vi "CONFOCAL MICROSCOPE - ( POSITION CURSOR).vi"() -> ()   [LabVIEW 2025]
uses:
  <vilib>/Analysis/1siggen.llb/Ramp Pattern by Samples.vi
  <vilib>/DAQmx/write.llb/DAQmx Write (Analog 1D Wfm NChan NSamp).vi
  <vilib>/DAQmx/read.llb/DAQmx Read (Counter 1D U32 1Chan NSamp).vi
  <vilib>/DAQmx/create/channels.llb/DAQmx Create Channel (AO-Voltage-Basic).vi
  <vilib>/DAQmx/configure/timing.llb/DAQmx Timing (Sample Clock).vi
  <vilib>/DAQmx/configure/events/hardwareSignals.llb/DAQmx Export Signal (Most Signals).vi
  <vilib>/DAQmx/miscellaneous.llb/DAQmx Fill In Error Info.vi
  <vilib>/DAQmx/create/channels.llb/DAQmx Create Channel (CI-Count Edges).vi
  <vilib>/Analysis/NI_AALBase.lvlib
panel:
  out "64bit integer":i64[](array[numeric])
  in  "volts":dbl=1.0 format="%_2f"
  in  "pixels":dbl
  out "transposed array":dbl[][](array[numeric])
  out "Intensity Graph":dbl[][](graph)
  out "Min Voltage (V)":dbl
  out "Max Voltage (V)":dbl
  in  "Dwell time (s)":dbl
  in  "Sample mode":i32(ring)=10178 items=["Finite Samples"=10178, "Continuous Samples"=10123, "Hardware Timed Single Point"=12522]
  out "appended array":dbl[][](array[numeric])
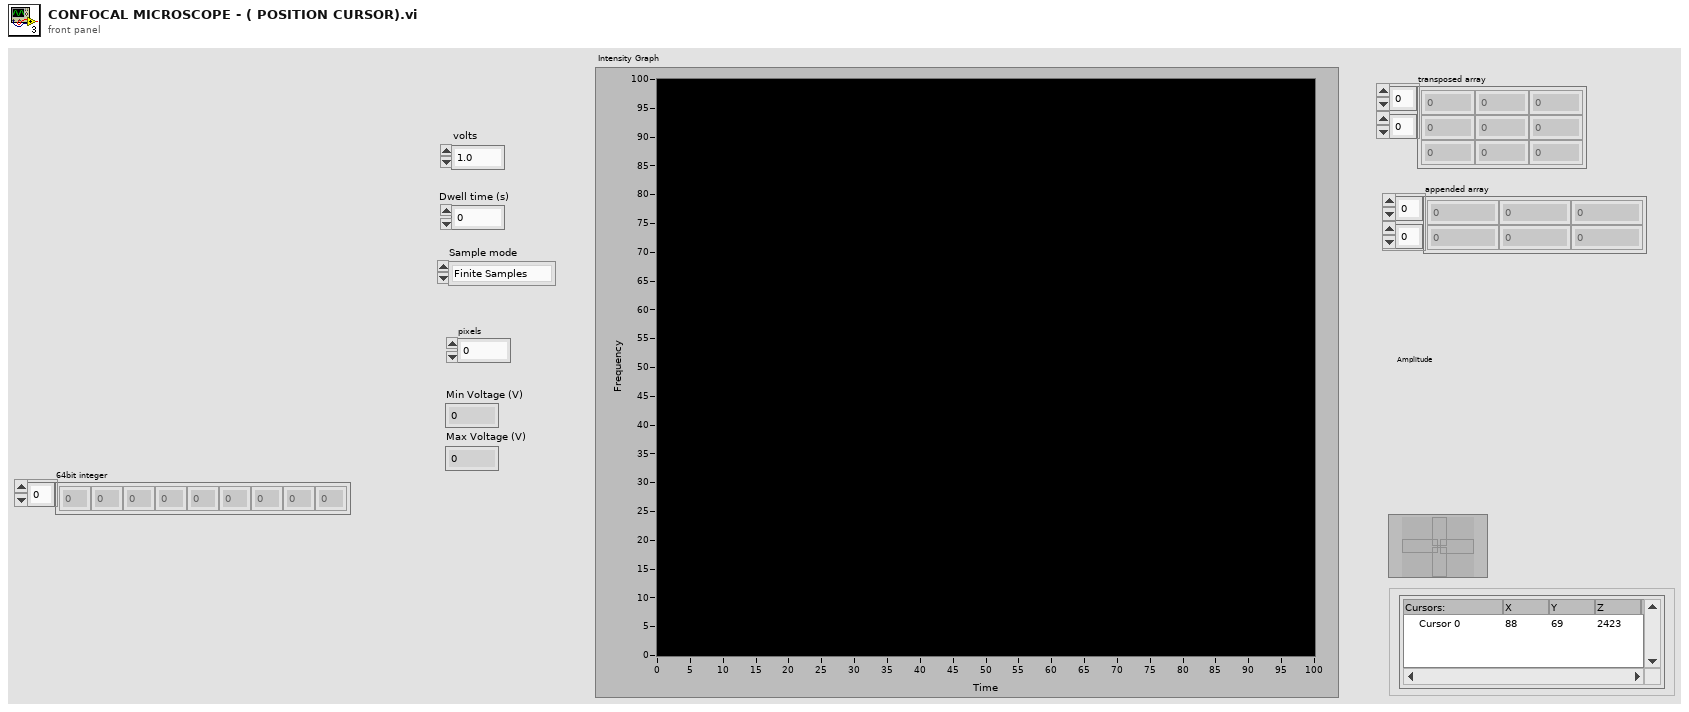
[diagram p1: front panel]
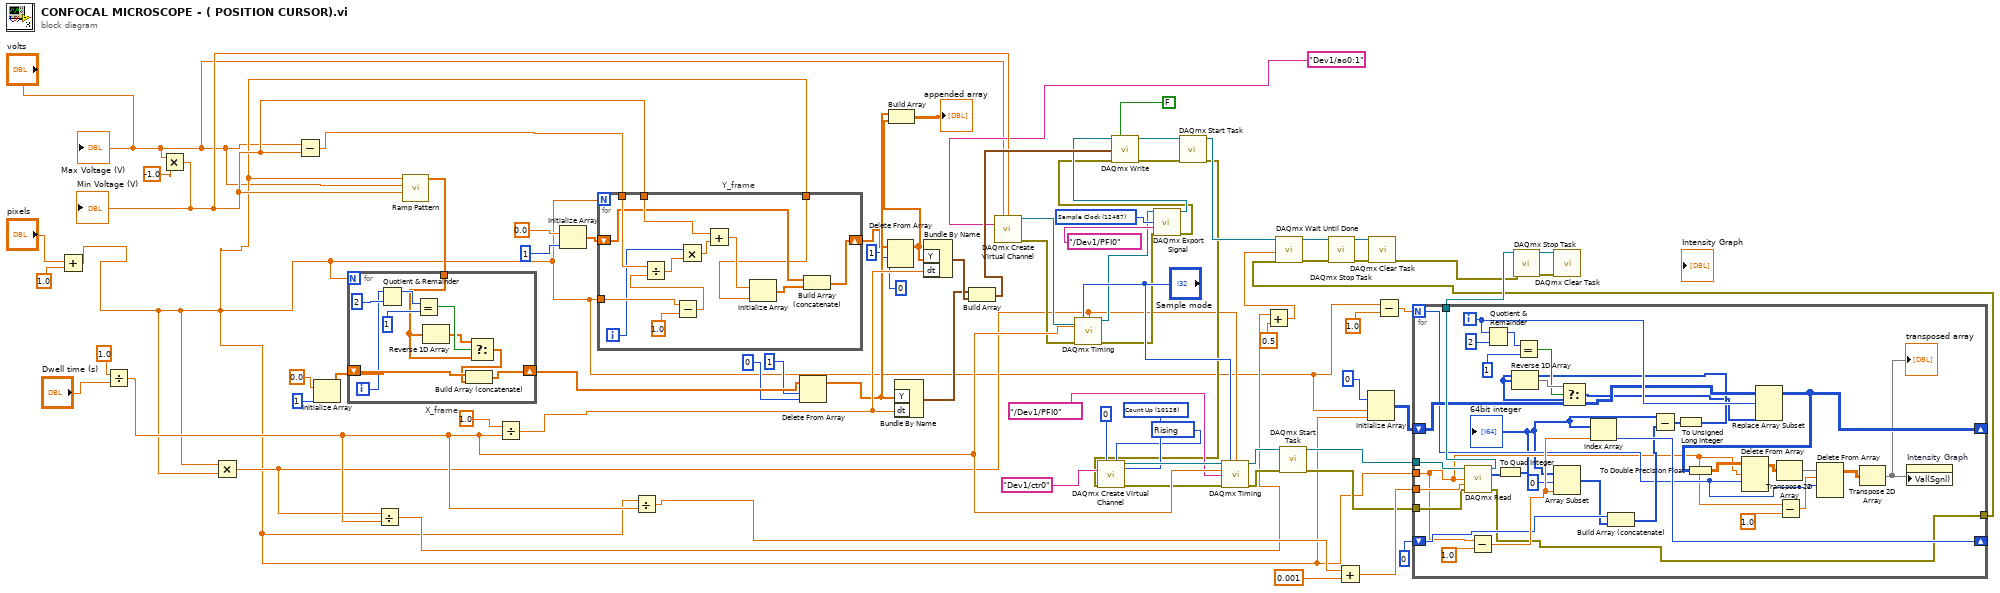
[diagram p0: block diagram]
diagram:
  w45 = 12487 items=["AI Convert Clock"=12484, "10MHz Reference Clock"=12536, "20MHz Timebase Clock"=12486, "Sample Clock"=12487, "Advance Trigger"=12488, "Reference Trigger"=12490, "Start Trigger"=12491, "Advance Complete Event"=12492, "AI Hold Complete Event"=12493, "Counter Output Event"=12494, "Change Detection Event"=12511, "Watchdog Timer Expired Event"=12512] ("signal")
  w50 = 10280 items=["Rising"=10280, "Falling"=10171] ("edge")
  w51 = 10128 items=["Count Up"=10128, "Count Down"=10124, "Externally Controlled"=10326] ("count direction")
  n1 = Add(x="pixels", y=1.0) -> (x+y=w2:dbl)
  n2 = Divide(x=1.0, y="Dwell time (s)") -> (x/y=w30:dbl)
  n3 = Multiply(x="volts", y=-1.0) -> (x*y=w6:dbl)
  "Min Voltage (V)" <- w6
  n4 = Multiply(x=w2, y=w2) -> (x*y=w11:dbl)
  n5 = Subtract(x="volts", y=w6) -> (x-y=w47:dbl)
  n6 = Initialize Array(0.0 ("element"), 1 ("dimension size")) -> (w58:dbl[])
  n7 = Divide(x=w11, y=w30) -> (x/y=w10:dbl)
  n8 = call-poly <vilib>:"Ramp Pattern.vi"("start"=w6, "end"="volts", "samples"=w2) -> ("Ramp Pattern"=w74:dbl[])  [unwired: 7 in, 1 out]
  n9 = for "X_frame" {
    N: w2 -> [_]
    shift-right: [w87] -> w41
    shift-left: w58 -> [w88]
    tunnel: w74 -> [w81]
    i -> [w82]
    n10 = Quotient & Remainder(x=w82, y=2) -> (x-y*floor(x/y)=w85:i32)  [unwired: 1 out]
    n11 = Equal?(x=w85, y=1) -> (x = y?=w83:bool)
    n12 = Reverse 1D Array(array=w81) -> (reversed array=w80:dbl[])
    n13 = Select(t=w80, s=w83, f=w81) -> (s? t:f=w79:dbl[])
    n14 = Build Array (concatenate)(w88, w79) -> (w87:dbl[])
  }
  n15 = Divide(x=1.0, y=w30) -> (x/y=w60:dbl)
  n16 = Initialize Array(0.0 ("element"), 1 ("dimension size")) -> (w59:dbl[])
  n17 = for "Y_frame" {
    N: w2 -> [_]
    tunnel: w2 -> [w101]
    tunnel: w47 -> [w99]
    tunnel: w6 -> [w94]
    tunnel: w2 -> [w89]
    shift-right: [w90] -> w37
    shift-left: w59 -> [w91]
    i -> [w96]
    n18 = Subtract(x=w101, y=1.0) -> (x-y=w98:dbl)
    n19 = Divide(x=w99, y=w98) -> (x/y=w97:dbl)
    n20 = Multiply(x=w96, y=w97) -> (x*y=w95:dbl)
    n21 = Add(x=w94, y=w95) -> (x+y=w93:dbl)
    n22 = Initialize Array(w93, w89) -> (w92:dbl[])
    n23 = Build Array (concatenate)(w91, w92) -> (w90:dbl[])
  }
  n24 = Divide(x=w2, y=w30) -> (x/y=w26:dbl)
  n25 = Delete From Array "Delete From Array"(array=w41, length=1, index=0) -> (array with subset deleted=w38:dbl[])  [unwired: 1 out]
  n26 = Delete From Array "Delete From Array"(array=w37, length=1, index=0) -> (array with subset deleted=w31:dbl[])  [unwired: 1 out]
  n27 = Build Array(w38, w31) -> (→"appended array":dbl[][])
  n28 = Bundle By Name("Y"=w38, "dt"=w60) -> (w61:waveform(dbl))  [unwired: 1 in]
  n29 = Bundle By Name("Y"=w31, "dt"=w60) -> (w62:waveform(dbl))  [unwired: 1 in]
  n30 = Build Array(w61, w62) -> (w64:waveform(dbl)[])
  n31 = call-poly <vilib>:"DAQmx Create Virtual Channel.vi"("maximum value"="volts", "minimum value"=w6, "physical channels"="Dev1/ao0:1" ("Galvo mirror path")) -> ("task out"=w63:refnum<k21>, "error out"=w24:errorcluster)  [unwired: 11 in]
  n32 = call-poly <vilib>:"DAQmx Timing.vi"("task/channels in"=w63, "sample mode"="Sample mode", "samples per channel"=w11, "rate"=w30, "error in"=w24) -> ("task out"=w43:refnum<k21>, "error out"=w23:errorcluster)  [unwired: 9 in]
  n33 = call-poly <vilib>:"DAQmx Export Signal.vi"("task/channels in"=w43, "signal"=w45, "output terminal"=tag "/Dev1/PFI0", "error in"=w23) -> ("task out"=w42:refnum<k21>, "error out"=w22:errorcluster)  [unwired: 10 in]
  n34 = call-poly <vilib>:"DAQmx Write.vi"("task/channels in"=w42, "auto start"=FALSE, "data"=w64, "error in"=w22) -> ("task out"=w65:refnum<k21>, "error out"=w21:errorcluster)  [unwired: 9 in, 1 out]
  n35 = call <vilib>:"DAQmx Start Task.vi"("task/channels in"=w65, "error in"=w21) -> ("task out"=w72:refnum<k21>, "error out"=w18:errorcluster)  [unwired: 12 in]
  n36 = call-poly <vilib>:"DAQmx Create Virtual Channel.vi"("initial count"=u32 0, "count direction"=w51, "edge"=w50, "counter"="Dev1/ctr0" ("Counter path"), "error in"=w18) -> ("task out"=w67:refnum<k21>, "error out"=w20:errorcluster)  [unwired: 9 in]
  n37 = call-poly <vilib>:"DAQmx Timing.vi"("task/channels in"=w67, "sample mode"="Sample mode", "samples per channel"=w11, "rate"=w30, "source"=tag "/Dev1/PFI0", "error in"=w20) -> ("task out"=w68:refnum<k21>, "error out"=w19:errorcluster)  [unwired: 8 in]
  n38 = Add(x=w10, y=0.5) -> (x+y=w8:dbl)
  n39 = call <vilib>:"DAQmx Start Task.vi"("task/channels in"=w68, "error in"=w19) -> ("task out"=w69:refnum<k21>, "error out"=w13:errorcluster)  [unwired: 12 in]
  n40 = Add(x=w26, y=0.001) -> (x+y=w32:dbl)
  n41 = Initialize Array(u32 0 ("element"), w2, w2) -> (w71:u32[][])
  n42 = Subtract(x=w2, y=1.0) -> (x-y=w28:dbl)
  n43 = for {
    N: w28 -> [w108]
    tunnel: w2 -> [w104]
    tunnel: w32 -> [w135]
    tunnel: w69 -> [w134]
    shift-right: [w117] -> _
    shift-left: w71 -> [w120]
    tunnel: [w129] -> w25
    shift-right: [w126] -> _
    shift-left: u64 0 ("Numeric") -> [w124]
    tunnel: w13 -> [w115]
    tunnel: [w114] -> w12
    i -> [w121]
    n44 = call-poly <vilib>:"DAQmx Read.vi"("task/channels in"=w134, "number of samples per channel"=w104, "timeout"=w135, "error in"=w115) -> ("task out"=w129:refnum<k21>, "data"=w116:u32[], "error out"=w114:errorcluster)  [unwired: 9 in]
    n45 = Subtract(x=w104, y=1.0) -> (x-y=w125:dbl)
    n46 = Quotient & Remainder(x=w121, y=2) -> (x-y*floor(x/y)=w132:i32)  [unwired: 1 out]
    n47 = To Quad Integer(1:w116) -> (0:w102:i64[])
    "64bit integer" <- w102
    n48 = Equal?(x=w132, y=1) -> (x = y?=w128:bool)
    n49 = Array Subset "Array Subset"(array=w102, index=0, length=w125) -> (w103:i64[])
    n50 = Index Array "Index Array"(array=w102, index=w125) -> (element=w126:i64)
    n51 = Build Array (concatenate) "Build Array"(w124, w103) -> (w123:u64[])
    n52 = Subtract(x=w102, y=w123) -> (x-y=w122:u64[])
    n53 = To Unsigned Long Integer(number=w122) -> (unsigned 32bit integer=w119:u32[])
    n54 = Reverse 1D Array(array=w119) -> (reversed array=w130:u32[])
    n55 = Select(t=w130, s=w128, f=w119) -> (s? t:f=w118:u32[])
    n56 = Replace Array Subset "Replace Array Subset"(array=w120, new element=w118, index (row)=w121) -> (w117:u32[][])  [unwired: 1 in]
    n57 = To Double Precision Float(number=w117) -> (double precision float=w113:dbl[][])
    n58 = Delete From Array(array=w113, length=w104, index (row)=w108) -> (array with subset deleted=w112:dbl[][])  [unwired: 1 in, 1 out]
    n59 = Transpose 2D Array(2D array=w112) -> (transposed array=w111:dbl[][])
    n60 = Subtract(x=w104, y=1.0) -> (x-y=w109:dbl)
    n61 = Delete From Array(array=w111, length=w109, index (row)=w108) -> (array with subset deleted=w107:dbl[][])  [unwired: 1 in, 1 out]
    n62 = Transpose 2D Array(2D array=w107) -> (transposed array=w106:dbl[][])
    "transposed array" <- w106
    n63 = property on="Intensity Graph" class="IntGraph (strict)"("Val(Sgnl)"=w106) -> ()  [unwired: 2 in, 2 out]
  }
  n64 = call <vilib>:"DAQmx Wait Until Done.vi"("task/channels in"=w72, "timeout (sec)"=w8, "error in"=w12) -> ("task out"=w73:refnum<k21>, "error out"=w17:errorcluster)  [unwired: 11 in]
  n65 = call <vilib>:"DAQmx Stop Task.vi"("task/channels in"=w73, "error in"=w17) -> ("task out"=w66:refnum<k21>, "error out"=w16:errorcluster)  [unwired: 12 in]
  n66 = call <vilib>:"DAQmx Clear Task.vi"("task in"=w66, "error in"=w16) -> ("error out"=w15:errorcluster)  [unwired: 13 in]
  n67 = call <vilib>:"DAQmx Stop Task.vi"("task/channels in"=w25, "error in"=w15) -> ("task out"=w75:refnum<k21>, "error out"=w14:errorcluster)  [unwired: 12 in]
  n68 = call <vilib>:"DAQmx Clear Task.vi"("task in"=w75, "error in"=w14) -> ()  [unwired: 13 in, 1 out]
  "Max Voltage (V)" <- "volts"
